vi "Enumerate Task Types.vi"() -> (2 "All Task Types":refnum<class "Task.lvclass">[](array[class]))   [LabVIEW 2020, in "Volatus.lvlib"]
uses:
  Volatus.lvlib
  Task/Task.lvclass
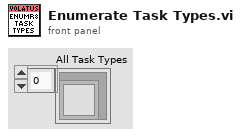
[diagram p1: front panel]
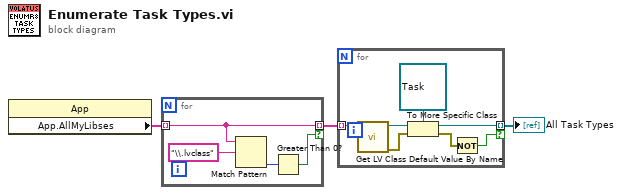
[diagram p0: block diagram]
diagram:
  n1 = property class="App"() -> ("App.AllMyLibses"=w3:string[])  [unwired: 2 in, 2 out]
  n2 = for {
    tunnel: w3 -> [w6] mode=indexing
    tunnel: [w6] -> w2 mode=indexing if=w4
    n3 = Match Pattern(string=w6, regular expression="\\.lvclass") -> (offset past match=w5:i32)  [unwired: 1 in, 3 out]
    n4 = Greater Than 0?(x=w5) -> (x > 0?=w4:bool)
  }
  n5 = for {
    tunnel: w2 -> [w14] mode=indexing
    tunnel: [w10] -> w1 mode=indexing if=w8
    n6 = call <vilib>:"Get LV Class Default Value By Name.vi"("class name"=w14) -> ("error out"=w11:errorcluster, "object"=w13:refnum<class>)  [unwired: 9 in]
    n7 = To More Specific Class(target class=refnum<class "Task.lvclass"> refnum ("Volatus:Task"), reference=w13, error in=w11) -> (specific class reference=w10:refnum<class "Task.lvclass">, error out=w9:errorcluster)
    n8 = Not(x=w9) -> (.not. x?=w8:bool)
  }
  "All Task Types" <- w1
